vi "addNewRun.vi"(8 "error in (no error)":errorcluster, 10 "New Run":refnum<class "xwpfRun.lvclass">, 11 "xwpfParagraph in":refnum<class "xwpfParagraph.lvclass">) -> (0 "error out":errorcluster, 3 "xwpfParagraph out":refnum<class "xwpfParagraph.lvclass">)   [LabVIEW 2017, in "Word_Specific.lvlib" / "xwpfParagraph.lvclass"]
uses:
  xwpfParagraph.lvclass
  xwpfRun/xwpfRun.lvclass
  xwpfRun/xwpfRun.lvclass/xwpfRun.ctl
  xwpfParagraph.lvclass/xwpfParagraph.ctl
  C:/Users/Neo/Desktop/Dev_Tools_BR/LabVIEW_NPOI/lib/NPOI 2.1.1/NPOI.OOXML.dll
  lib/NPOI 2.1.1/NPOI.OOXML.dll
  xwpfRun/Get Run Ref.vi
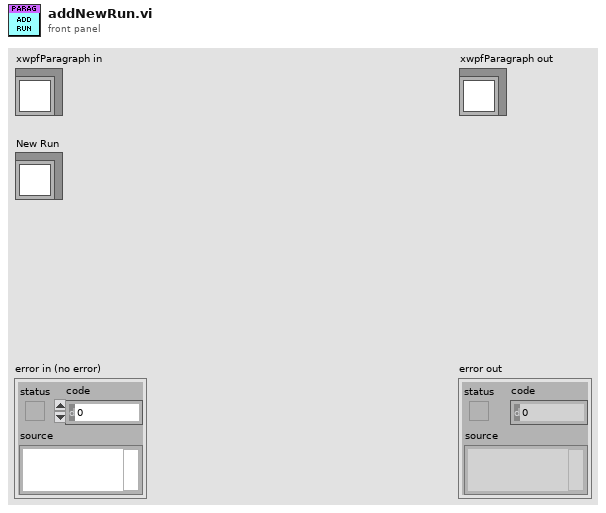
[diagram p1: front panel]
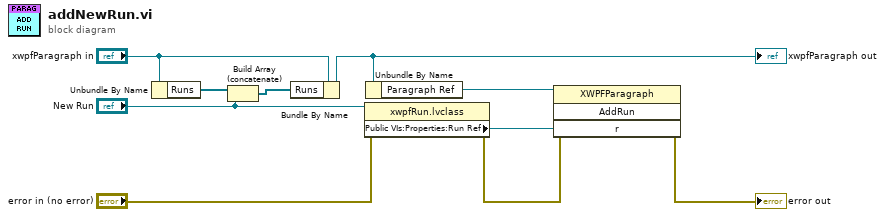
[diagram p0: block diagram]
diagram:
  n1 = Unbundle By Name("xwpfParagraph in") -> ("Runs"=w10:refnum<class "xwpfRun.lvclass">[])
  n2 = Build Array (concatenate)(w10, "New Run") -> (w9:refnum<class "xwpfRun.lvclass">[])
  n3 = Bundle By Name(cluster="xwpfParagraph in", "Runs"=w9) -> (w5:refnum<class "xwpfParagraph.lvclass">)
  "xwpfParagraph out" <- w5
  n4 = property class="xwpfRun.lvclass"(reference="New Run", error in="error in (no error)") -> (error out=w2:errorcluster, "Public VIs:Properties:Run Ref"=w6:refnum<k24>)  [unwired: 1 out]
  n5 = Unbundle By Name(w5) -> ("Paragraph Ref"=w7:refnum<k24>)
  n6 = invoke class="XWPFParagraph" method="AddRun"(reference=w7, error in=w2, "r"=w6) -> (error out=→"error out":errorcluster)  [unwired: 1 in, 3 out]
